vi "GD.vi"(1 "BMP File Path":path, 2 "XML File Path":path) -> (0 "vi refnum":refnum<vi>)   [LabVIEW 2017]
panel:
  in  "out":i8[](array[numeric])
  in  "XML File Path 2":path
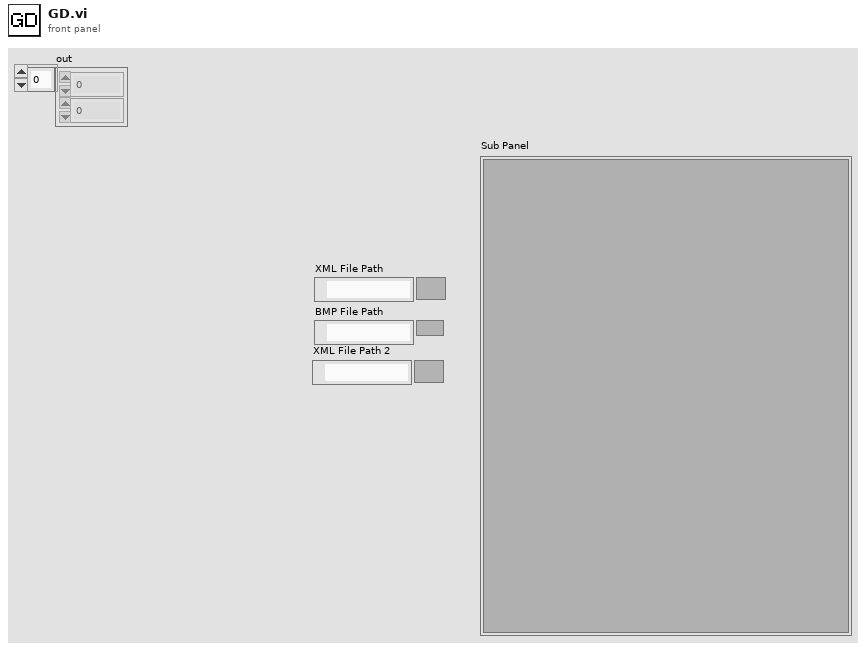
[diagram p1: front panel]
types:
  T1 = cluster{"node text":string, cluster{"[0]":i32, "[1]":i32}, i32, bool, bool, cluster{"[0]":u32, "[1]":u32}[], i32, "String":string, bool, i32, i32, i32, "node text":string}[]
  T2 = cluster{refnum<vi>, bool, i32, i32, "node text":string}[]
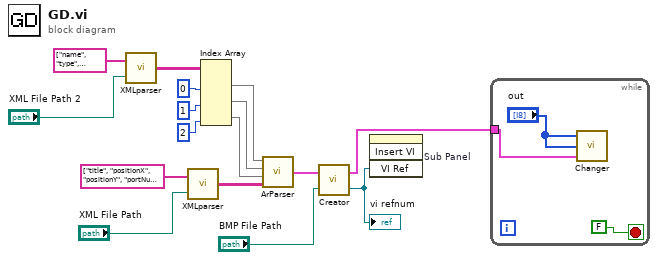
[diagram p0: block diagram]
diagram:
  n1 = call "XMLparser.vi"("XML File Path"="XML File Path 2", "Array"=string[] ["name", "type", "class"]) -> ("toArrayParser"=w10:string[][])
  n2 = call "XMLparser.vi"("XML File Path"="XML File Path", "Array"=string[] ["title", "positionX", "positionY", "portNum", "portType", "colorTrue", "colorFalse", "type", "bitNum", "minRange", "difRange"]) -> ("toArrayParser"=w3:string[][])
  n3 = Index Array(array=w10, index (col) #1=0 ("index (row)"), index (col) #2=1 ("index (row)"), index (col) #3=2 ("index (row)")) -> (element #1=w6:string[], element #2=w5:string[], element #3=w4:string[])  [unwired: 3 in]
  n4 = call "ArParser.vi"("from\nXMLparser"=w3, "IndicatorClasses"=w4, "IndicatorTypes"=w5, "IndicatorNames"=w6) -> ("toCreator"=w2:T1)
  n5 = call "Creator.vi"("BMP File Path"="BMP File Path", "toCreator"=w2) -> ("subvi"=w15:refnum<vi>, "toChanger"=w1:T2)
  "vi refnum" <- w15
  n6 = invoke on="Sub Panel" class="SubPnl" method="Insert VI"("VI Ref"=w15) -> ()  [unwired: 3 in, 4 out]
  n7 = while {
    tunnel: w1 -> [w18]
    stop <- FALSE stop-if-true
    n8 = call "Changer.vi"("toChanger"=w18, "out"="out", "in"="out") -> ()
  }
